vi "AirHeater.vi"(1 "Controll Signal":dbl) -> (0 "Temperature [C]":dbl)   [LabVIEW 2025]
panel:
  # "Air Heater"
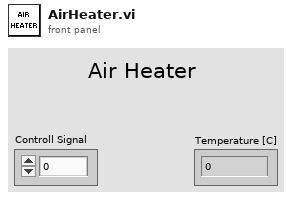
[diagram p1: front panel]
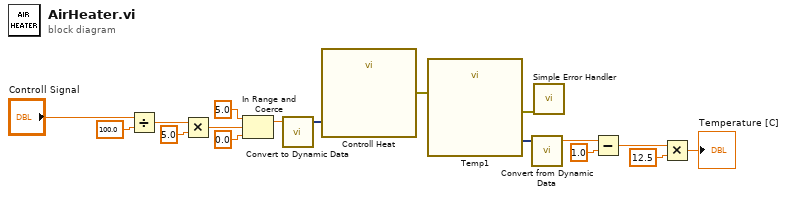
[diagram p0: block diagram]
diagram:
  n1 = Divide(x="Controll Signal", y=100.0) -> (x/y=w15:dbl)
  n2 = Multiply(x=w15, y=5.0) -> (x*y=w4:dbl)
  n3 = In Range and Coerce(upper limit=5.0, x=w4, lower limit=0.0) -> (coerced(x)=w1:dbl)  [unwired: 1 out]
  n4 = call "Convert to Dynamic Data"("Double"=w1) -> ("Dynamic Data Type"=w7:dynamicdata)  [unwired: 3 in]
  n5 = call "Controll Heat"("data"=w7) -> ("error out"=w6:errorcluster)  [unwired: 17 in, 1 out]
  n6 = call "Temp1"("error in"=w6) -> ("data"=w8:dynamicdata, "error out"=w5:errorcluster)  [unwired: 16 in, 1 out]
  n7 = call "Convert from Dynamic Data"("Dynamic Data Type"=w8) -> ("Scalar"=w9:dbl)  [unwired: 3 in]
  n8 = call <vilib>:"Simple Error Handler.vi"("error in (no error)"=w5) -> ()  [unwired: 4 in, 5 out]
  n9 = Subtract(x=w9, y=1.0) -> (x-y=w10:dbl)
  n10 = Multiply(x=w10, y=12.5) -> (x*y=→"Temperature [C]":dbl)
